vi "6 motor arcade drive.vi"(8 "Y Axis":dbl, 11 "X Axis":dbl) -> ()   [LabVIEW 2017]
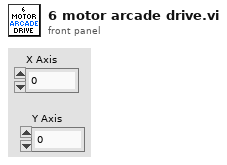
[diagram p1: front panel]
types:
  T1 = typedef "WPI_MotorControlDeviceRef.ctl" = cluster{"DeviceStatus":errorcluster, "Type":T2, "PWM":cluster{"PWM Channel":T3, "DeadBand":T4}, "CAN":cluster{"Device Number":u8, "SetOutput VI Ref":variant, "GetOutput VI Ref":variant, "Enable VI Ref":variant, "Disable VI Ref":variant, "Data":variant}, "Invert":bool, "DIO PWM":cluster{"PWM \"Enable\" Channel":T3, "DIOChannel":T5, "PWM Rate":dbl}}
  T2 = typedef "WPI_MotorControlType.ctl" = enum16{"PWM", "CAN", "DIO PWM"}
  T3 = typedef "FPGA_DIOPWMChannel.ctl" = enum8{"PWM 0", "PWM 1", "PWM 2", "PWM 3", "PWM 4", "PWM 5", "PWM 6", "PWM 7", "PWM 8", "PWM 9", "PWM MXP 0", "PWM MXP 1", "PWM MXP 2", "PWM MXP 3", "PWM MXP 4", "PWM MXP 5", "PWM MXP 6", "PWM MXP 7", "PWM MXP 8", "PWM MXP 9", "Invalid"}
  T4 = typedef "WPI_PWMDeadband.ctl" = cluster{"Name":string, "maxPositivePwm":i32, "minPositivePwm":i32, "centerPwm":i32, "maxNegativePwm":i32, "minNegativePwm":i32, "angularRange":u16}
  T5 = typedef "FPGA_DIOChannel.ctl" = enum8{"DIO 0", "DIO 1", "DIO 2", "DIO 3", "DIO 4", "DIO 5", "DIO 6", "DIO 7", "DIO 8", "DIO 9", "DIO MXP 0", "DIO MXP 1", "DIO MXP 2", "DIO MXP 3", "DIO MXP 4", "DIO MXP 5", "DIO MXP 6", "DIO MXP 7", "DIO MXP 8", "DIO MXP 9", "DIO MXP 10", "DIO MXP 11", "DIO MXP 12", "DIO MXP 13", "DIO MXP 14", "DIO MXP 15", "SPI Port CS1", "SPI Port CS2", "SPI Port CS3", "SPI Port MISO", "SPI Port MOSI", "Invalid"}
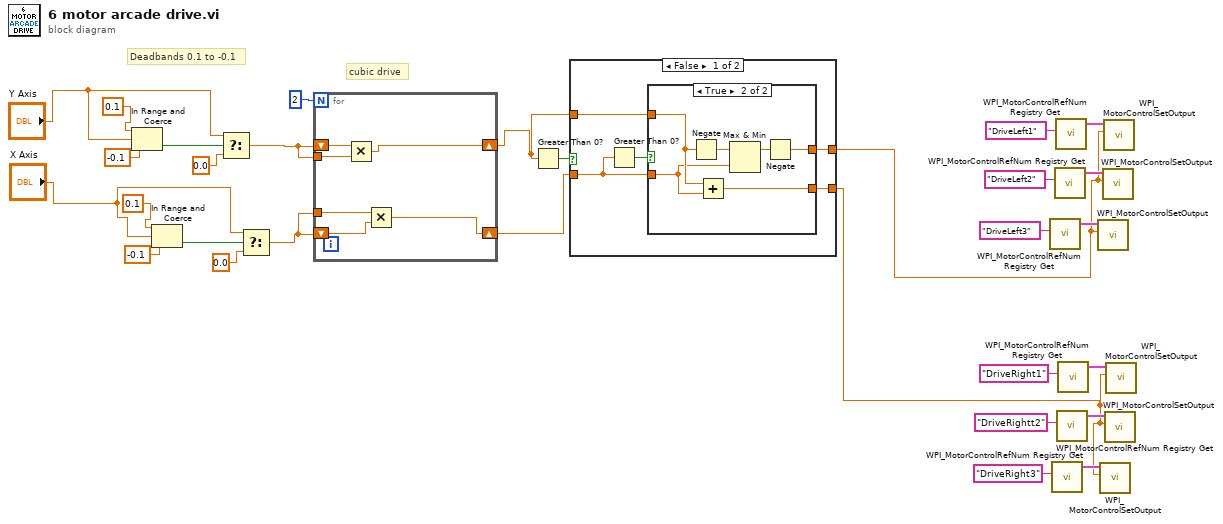
[diagram p0: block diagram]
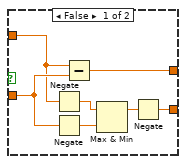
[diagram p2: hidden frame]
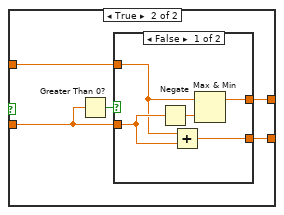
[diagram p3: hidden frame]
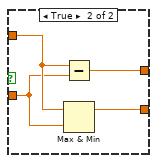
[diagram p4: hidden frame]
diagram:
  # "cubic drive"
  # "Deadbands 0.1 to -0.1"
  n1 = In Range and Coerce(upper limit=0.1, x="Y Axis", lower limit=-0.1) -> (In Range?=w15:bool)  [unwired: 1 out]
  n2 = In Range and Coerce(upper limit=0.1, x="X Axis", lower limit=-0.1) -> (In Range?=w8:bool)  [unwired: 1 out]
  n3 = Select(t="Y Axis", s=w15, f=0.0) -> (s? t:f=w5:dbl)
  n4 = Select(t="X Axis", s=w8, f=0.0) -> (s? t:f=w4:dbl)
  n5 = for {
    N: 2 -> [_]
    shift-right: [w31] -> w3
    shift-left: w5 -> [w36]
    shift-right: [w32] -> w2
    shift-left: w4 -> [w34]
    tunnel: w5 -> [w35]
    tunnel: w4 -> [w33]
    n6 = Multiply(x=w36, y=w35) -> (x*y=w31:dbl)
    n7 = Multiply(x=w33, y=w34) -> (x*y=w32:dbl)
  }
  n8 = Greater Than 0?(x=w3) -> (x > 0?=w18:bool)
  n9 = case shown="False" w18 {
    tunnel: w2 -> [w40 w58]
    tunnel: w3 -> [w39 w57]
    tunnel: [w38 w56] -> w17
    tunnel: [w37 w55] -> w16
    frame False {
      n10 = Greater Than 0?(x=w40) -> (x > 0?=w41:bool)
      n11 = case shown="True" w41 {
        tunnel: w40 -> [w48 w50]
        tunnel: w39 -> [w46 w51]
        tunnel: [w42 w52] -> w38
        tunnel: [w43 w49] -> w37
        frame False {
          n12 = Negate(x=w46) -> (-x=w47:dbl)
          n13 = Negate(x=w48) -> (-x=w45:dbl)
          n14 = Subtract(x=w46, y=w48) -> (x-y=w42:dbl)
          n15 = Max & Min(x=w47, y=w45) -> (max(x,y)=w44:dbl)  [unwired: 1 out]
          n16 = Negate(x=w44) -> (-x=w43:dbl)
        }
        frame True {
          n17 = Negate(x=w51) -> (-x=w54:dbl)
          n18 = Add(x=w51, y=w50) -> (x+y=w49:dbl)
          n19 = Max & Min(x=w54, y=w50) -> (max(x,y)=w53:dbl)  [unwired: 1 out]
          n20 = Negate(x=w53) -> (-x=w52:dbl)
        }
      }
    }
    frame True {
      n21 = Greater Than 0?(x=w58) -> (x > 0?=w59:bool)
      n22 = case shown="False" w59 {
        tunnel: w58 -> [w64 w66]
        tunnel: w57 -> [w61 w67]
        tunnel: [w62 w65] -> w56
        tunnel: [w60 w68] -> w55
        frame False {
          n23 = Negate(x=w64) -> (-x=w63:dbl)
          n24 = Add(x=w61, y=w64) -> (x+y=w60:dbl)
          n25 = Max & Min(x=w61, y=w63) -> (max(x,y)=w62:dbl)  [unwired: 1 out]
        }
        frame True {
          n26 = Subtract(x=w67, y=w66) -> (x-y=w65:dbl)
          n27 = Max & Min(x=w67, y=w66) -> (max(x,y)=w68:dbl)  [unwired: 1 out]
        }
      }
    }
  }
  n28 = call <vilib>:"WPI_MotorControlRefNum Registry Get.vi"("refnum name"="DriveLeft3") -> ("MotorControlDevRef"=w26:T1)  [unwired: 9 in, 1 out]
  n29 = call <vilib>:"WPI_MotorControlRefNum Registry Get.vi"("refnum name"="DriveRight3") -> ("MotorControlDevRef"=w23:T1)  [unwired: 9 in, 1 out]
  n30 = call <vilib>:"WPI_MotorControlRefNum Registry Get.vi"("refnum name"="DriveLeft2") -> ("MotorControlDevRef"=w27:T1)  [unwired: 9 in, 1 out]
  n31 = call <vilib>:"WPI_MotorControlRefNum Registry Get.vi"("refnum name"="DriveLeft1") -> ("MotorControlDevRef"=w30:T1)  [unwired: 9 in, 1 out]
  n32 = call <vilib>:"WPI_MotorControlRefNum Registry Get.vi"("refnum name"="DriveRightt2") -> ("MotorControlDevRef"=w22:T1)  [unwired: 9 in, 1 out]
  n33 = call <vilib>:"WPI_MotorControlRefNum Registry Get.vi"("refnum name"="DriveRight1") -> ("MotorControlDevRef"=w19:T1)  [unwired: 9 in, 1 out]
  n34 = call <vilib>:"WPI_MotorControlSetOutput.vi"("Output"=w17, "MotorControlDevRef"=w26) -> ()  [unwired: 7 in, 3 out]
  n35 = call <vilib>:"WPI_MotorControlSetOutput.vi"("Output"=w16, "MotorControlDevRef"=w23) -> ()  [unwired: 7 in, 3 out]
  n36 = call <vilib>:"WPI_MotorControlSetOutput.vi"("Output"=w17, "MotorControlDevRef"=w27) -> ()  [unwired: 7 in, 3 out]
  n37 = call <vilib>:"WPI_MotorControlSetOutput.vi"("Output"=w17, "MotorControlDevRef"=w30) -> ()  [unwired: 7 in, 3 out]
  n38 = call <vilib>:"WPI_MotorControlSetOutput.vi"("Output"=w16, "MotorControlDevRef"=w22) -> ()  [unwired: 7 in, 3 out]
  n39 = call <vilib>:"WPI_MotorControlSetOutput.vi"("Output"=w16, "MotorControlDevRef"=w19) -> ()  [unwired: 7 in, 3 out]
